vi "_DumpTelemetry.vi"(8 "error in (no error)":errorcluster, 10 "Telemetry":refnum<k21>, 11 "MPU in":refnum<class "MPU.lvclass">) -> (3 "MPU out":refnum<class "MPU.lvclass">)   [LabVIEW 2018, in "Modbus_Processing_Unit.lvlib" / "MPU.lvclass"]
uses:
  MPU.lvclass
  MPU.lvclass/MPU.ctl
  <vilib>/rvi/DataTransferAndStorage/Container/Common/niFpgaContainerExecOnDevCompGetState.vi
  <vilib>/rvi/Emulation/niFpgaEmulationIsFPGAContextNoSignature.vi
  <vilib>/rvi/Emulation/niFpgaSctlEmulationGetInTimedLoop.vi
  <vilib>/rvi/errors/niFpgaSetErrorForExecOnDevCompSimple.vi
  <vilib>/rvi/eio/common/nirviEmuReportErrorAndStop.vi
  <vilib>/rvi/DataTransferAndStorage/Container/Common/niFpgaContainerGetUniqueNameForEmu.vi
  <vilib>/rvi/FIFO/Fifo_Resource/nirvififoEmulationSetSize.vi
  <vilib>/rvi/FIFO/Fifo_Resource/nirviFifoEmulationQueueMgr.vi
  <instcachedir>/0/nirviFifoEmulationQueueMgr_E5CAEC123FF24DC58D834DCA3CDAA9B5.lvgen/nirviFifoEmulationQueueMgr_E5CAEC123FF24DC58D834DCA3CDAA9B5_001.vi
  <vilib>/rvi/FIFO/Fifo_Resource/nirvififoEmulationDetermineInputValidOut.vi
  <vilib>/rvi/FIFO/Fifo_Resource/nirvififoEmulationCreateLock.vi
  <vilib>/rvi/Emulation/niFpgaProcessEmulError.vi
  <vilib>/rvi/FIFO/Fifo_Resource/nirvififoEmulationObtainLock.vi
  <vilib>/rvi/FIFO/Fifo_Resource/nirvififoEmulationReleaseLock.vi
  <vilib>/rvi/occurrence/nirviWaitOnOccurrenceBase.vi
  <vilib>/rvi/errors/nirviReportUnexpectedCaseInternalError.vi
  <vilib>/rvi/errors/nirviReportUnexpectedCaseInternalError (U32).vi
  <vilib>/Utility/error.llb/Clear Errors.vi
  <vilib>/rvi/interface/RandomDataEmulation/niFpgaRandomDataHandleErrors.vi
  <vilib>/rvi/DataTransferAndStorage/Container/XNode/niFpgaContainer.xnode
  <vilib>/rvi/FIFO/Fifo_Resource/niFpgaFifoEmulationRefIn.vi
  Modbus_Processing_Unit.lvlib
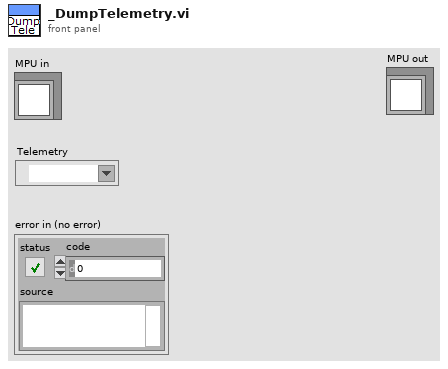
[diagram p1: front panel]
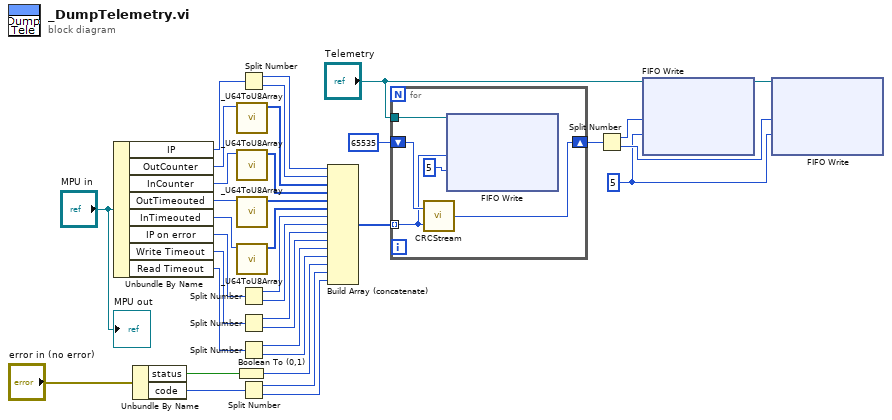
[diagram p0: block diagram]
diagram:
  w14 = 5 ("Timeout")
  n1 = Unbundle By Name("MPU in") -> ("IP"=w35:i16, "OutCounter"=w32:u64, "InCounter"=w30:u64, "OutTimeouted"=w27:u64, "InTimeouted"=w26:u64, "IP on error"=w24:i16, "Write Timeout"=w10:u16, "Read Timeout"=w9:u16)
  n2 = Unbundle By Name("error in (no error)") -> ("status"=w2:bool, "code"=w11:i32)
  n3 = Boolean To (0,1)(Boolean=w2) -> (0, 1=w1:i16)
  n4 = call "_U64ToU8Array.vi"("U64In"=w32) -> ("ArrayOut"=w31:u8[])  [unwired: 10 in]
  n5 = call "_U64ToU8Array.vi"("U64In"=w30) -> ("ArrayOut"=w29:u8[])  [unwired: 10 in]
  n6 = call "_U64ToU8Array.vi"("U64In"=w27) -> ("ArrayOut"=w28:u8[])  [unwired: 10 in]
  n7 = call "_U64ToU8Array.vi"("U64In"=w26) -> ("ArrayOut"=w25:u8[])  [unwired: 10 in]
  n8 = Split Number(x=w35) -> (hi(x)=w34:u8, lo(x)=w33:u8)
  n9 = Split Number(x=w24) -> (hi(x)=w23:u8, lo(x)=w22:u8)
  n10 = Split Number(x=w10) -> (hi(x)=w8:u8, lo(x)=w7:u8)
  n11 = Split Number(x=w9) -> (hi(x)=w6:u8, lo(x)=w5:u8)
  n12 = Split Number(x=w11) -> (hi(x)=w4:u16, lo(x)=w3:u16)
  n13 = Build Array (concatenate)(w34, w33, w31, w29, w28, w25, w23, w22, w8, w7, w6, w5, w1, w4, w3) -> (w20:u16[])
  n14 = for {
    tunnel: w20 -> [w38] mode=indexing
    shift-right: [w39] -> w18
    shift-left: u16 65535 -> [w40]
    tunnel: "Telemetry" -> [w37]
    n15 = call "CRCStream.vi"("Data"=w38, "Numeric in"=w40) -> ("Numeric out"=w39:u16)
    n16 = xnode ("FIFO Write")("Element"=w38, "Timeout"=5, "FIFO In"=w37) -> ()  [unwired: 2 out]
  }
  n17 = Split Number(x=w18) -> (hi(x)=w16:u8, lo(x)=w15:u8)
  n18 = xnode ("FIFO Write")("Element"=w16, "Timeout"=w14, "FIFO In"="Telemetry") -> ("FIFO Out"=w17:refnum<k21>)  [unwired: 1 out]
  n19 = xnode ("FIFO Write")("Element"=w15, "Timeout"=w14, "FIFO In"=w17) -> ()  [unwired: 2 out]
  "MPU out" <- "MPU in"
